vi "Add Transition.vi"(0 "State in":refnum<class "State.lvclass">, 5 "Target":string, 7 "Event":string, 9 "Type":string, 11 "error in (no error)":errorcluster, 12 "Action":T1) -> (4 "State out":refnum<class "State.lvclass">, 15 "error out":errorcluster)   [LabVIEW 2015, in "State.lvclass"]
uses:
  State.lvclass
  Typedefs/Tosca-Termination Condition Action.ctl
  State.lvclass/State.ctl
  Termination/Termination.lvclass/Termination.ctl
  Timeout/Timeout.lvclass/Timeout.ctl
  Termination/Write Action.vi
  Timeout/Write Link to.vi
  Termination/Termination.lvclass
  Timeout/Timeout.lvclass
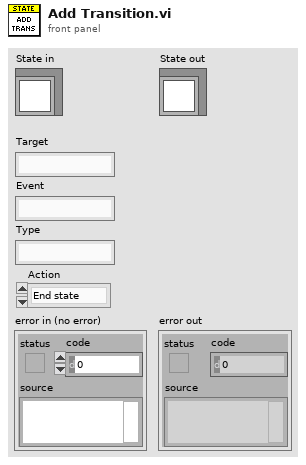
[diagram p1: front panel]
types:
  T1 = typedef "Tosca-Termination Condition Action.ctl" = enum16{"End state", "Complete state", "TTL only"}
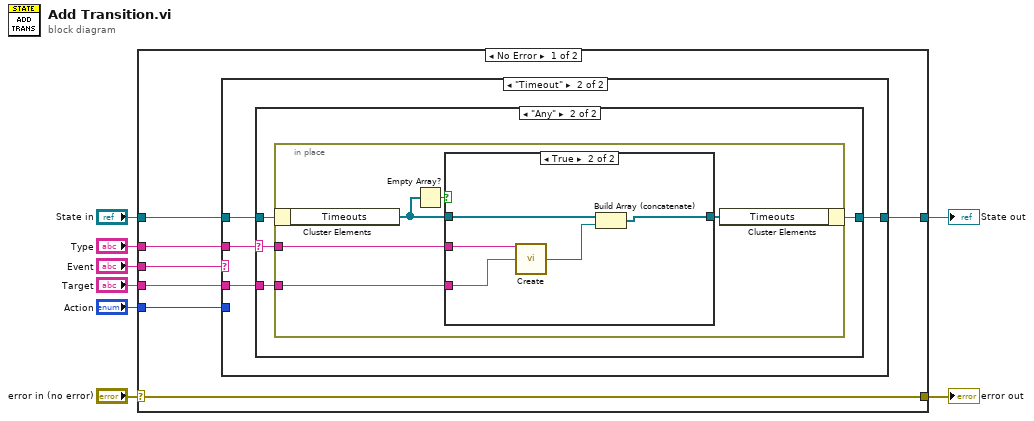
[diagram p0: block diagram]
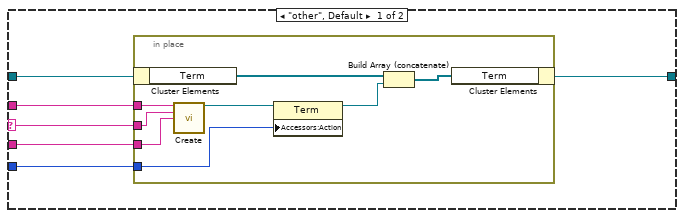
[diagram p2: hidden frame]
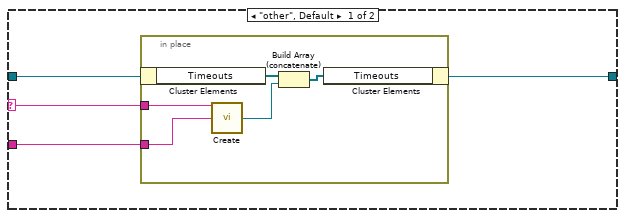
[diagram p3: hidden frame]
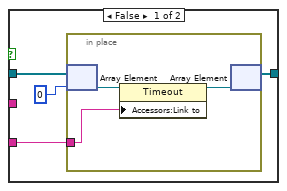
[diagram p4: hidden frame]
diagram:
  n1 = case shown="No Error" "error in (no error)" {
    selector: "error in (no error)" -> [w15 w65]
    tunnel: [w15 w65] -> w7
    tunnel: [w11 w64] -> w5
    tunnel: "State in" -> [w12 w64]
    tunnel: "Type" -> [w14 _]
    tunnel: "Event" -> [w13 _]
    tunnel: "Target" -> [w10 _]
    tunnel: "Action" -> [w9 _]
    frame No Error {
      n2 = case shown="\"Timeout\"" w13 {
        selector: w13 -> [w18 _]
        tunnel: w14 -> [w19 w33]
        tunnel: w12 -> [w21 w32]
        tunnel: [w20 w31] -> w11
        tunnel: w10 -> [w17 w30]
        tunnel: w9 -> [w16 _]
        frame "other", Default {
          n3 = in-place {
            in-place-border: w19 -> [w26]
            in-place-border: w18 -> [w25]
            in-place-border: w17 -> [w24]
            in-place-border: w16 -> [w22]
            n4 = in-place-cluster #1(w21) -> ("Term"=w29:refnum<class "Termination.lvclass">[])
            n5 = call "Create.vi"("Type"=w26, "Event"=w25, "Target"=w24) -> ("Termination"=w27:refnum<class "Termination.lvclass">)  [unwired: 12 in]
            n6 = property class="Term"(reference=w27, "Accessors:Action"=w22) -> (reference out=w23:refnum<class "Termination.lvclass">)  [unwired: 1 in, 1 out]
            n7 = Build Array (concatenate)(w29, w23) -> (w28:refnum<class "Termination.lvclass">[])
            n8 = in-place-cluster #1("Term"=w28) -> (w20:refnum<class "State.lvclass">)
          }
        }
        frame "Timeout" {
          n9 = case shown="\"Any\"" w33 {
            selector: w33 -> [w35 w43]
            tunnel: w32 -> [w37 w46]
            tunnel: [w36 w45] -> w31
            tunnel: w30 -> [w34 w44]
            frame "other", Default {
              n10 = in-place {
                in-place-border: w35 -> [w39]
                in-place-border: w34 -> [w38]
                n11 = in-place-cluster #2(w37) -> ("Timeouts"=w42:refnum<class "Timeout.lvclass">[])
                n12 = call "Create.vi"("Type"=w39, "Target"=w38) -> ("Timeout"=w40:refnum<class "Timeout.lvclass">)  [unwired: 13 in]
                n13 = Build Array (concatenate)(w42, w40) -> (w41:refnum<class "Timeout.lvclass">[])
                n14 = in-place-cluster #2("Timeouts"=w41) -> (w36:refnum<class "State.lvclass">)
              }
            }
            frame "Any" {
              n15 = in-place {
                in-place-border: w44 -> [w50]
                in-place-border: w43 -> [w47]
                n16 = in-place-cluster #3(w46) -> ("Timeouts"=w48:refnum<class "Timeout.lvclass">[])
                n17 = Empty Array?(array=w48) -> (empty?=w49:bool)
                n18 = case shown="True" w49 {
                  tunnel: w48 -> [w55 w63]
                  tunnel: [w53 w59] -> w51
                  tunnel: w50 -> [w52 w60]
                  tunnel: w47 -> [_ w61]
                  frame False {
                    n19 = in-place {
                      in-place-border: w52 -> [w56]
                      n20 = in-place-array #4(w55, 0) -> (w58:refnum<class "Timeout.lvclass">)
                      n21 = property class="Timeout"(reference=w58, "Accessors:Link to"=w56) -> (reference out=w57:refnum<class "Timeout.lvclass">)  [unwired: 1 in, 1 out]
                      n22 = in-place-array #4(w57) -> (w53:refnum<class "Timeout.lvclass">[])  [unwired: 1 out]
                    }
                  }
                  frame True {
                    n23 = call "Create.vi"("Type"=w61, "Target"=w60) -> ("Timeout"=w62:refnum<class "Timeout.lvclass">)  [unwired: 13 in]
                    n24 = Build Array (concatenate)(w63, w62) -> (w59:refnum<class "Timeout.lvclass">[])
                  }
                }
                n25 = in-place-cluster #3("Timeouts"=w51) -> (w45:refnum<class "State.lvclass">)
              }
            }
          }
        }
      }
    }
    frame Error {
    }
  }
  "error out" <- w7
  "State out" <- w5
